vi "Method.vi"(4 "Input B":refnum<class "Abs_Numeric.lvclass">, 5 "Input A":T1) -> (1 "Result":T1)   [LabVIEW 2021, in "Multiply_EXT.lvclass"]
uses:
  Multiply_EXT.lvclass
  Abs_Type.ctl
  Abs_Types/Extended Float/Abs_Extended Float.lvclass
  Abs_Types/Numeric/Abs_Numeric.lvclass
  C:/Users/Tim/Documents/LabVIEW/2021/Data Classes/Source/Functions/Support/Two Terminal/EXT/AbsFunc_Two Term_EXT.lvclass
  C:/Users/Tim/Documents/LabVIEW/2021/Data Classes/Source/Abs_Types/Extended Float/Abs_Extended Float.lvclass
  Support/Two Terminal/EXT/AbsFunc_Two Term_EXT.lvclass/AbsFunc_Two Term_EXT.ctl
  Support/Two Terminal/EXT/Properties/Write Numeric A.vi
  Support/Two Terminal/EXT/Properties/Write Numeric B.vi
  Multiply_EXT.lvclass/Multiply_EXT.ctl
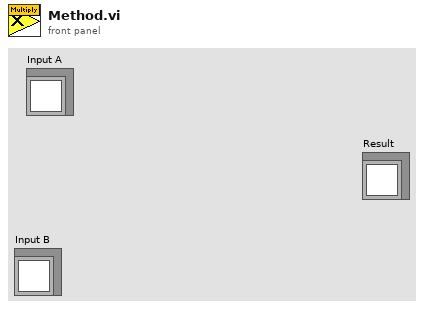
[diagram p1: front panel]
types:
  T1 = typedef "Multiply_EXT.lvclass/Abs_Type.ctl" = refnum<class "Abs_Extended Float.lvclass">
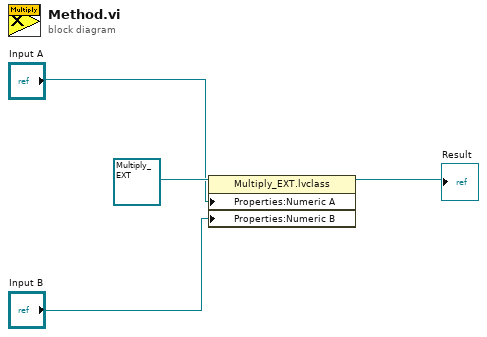
[diagram p0: block diagram]
diagram:
  n1 = property class="Multiply_EXT.lvclass"(reference=refnum<class "Multiply_EXT.lvclass"> refnum ("Functions.lvlib:Numeric.lvlib:Multiply.lvclass"), "Properties:Numeric A"="Input A", "Properties:Numeric B"="Input B") -> (reference out=→"Result":refnum<class "Multiply_EXT.lvclass">)  [unwired: 1 in, 1 out]
